vi "Initialize Transfer Groups.vi"(8 "error in (no error)":errorcluster, 10 "transfer group configurations":T1[](array[typedef]) {"transfers"."channels"."string offset" format="%d bytes"}, 11 "PXImc Transceiver in":refnum<class "DSF PXImc Transceiver.lvclass">=refnum) -> (0 "error out":errorcluster, 3 "PXImc Transceiver out":refnum<class "DSF PXImc Transceiver.lvclass">)   [LabVIEW 2017, in "DSF Core.lvlib" / "DSF PXImc Transceiver.lvclass"]
uses:
  DSF PXImc Transceiver.lvclass
  Typedefs/DSF Engine Transfer Group Configuration.ctl
  Typedefs/DSF Direction.ctl
  Typedefs/DSF Timing Info.ctl
  Typedefs/DSF Settings Info.ctl
  Typedefs/DSF Engine Transfer Configuration.ctl
  Typedefs/DSF Byte Order.ctl
  Typedefs/DSF Engine Channel Configuration.ctl
  Typedefs/DSF Data Type.ctl
  Typedefs/DSF Timeout Behavior.ctl
  PXImc Group Data.ctl
  PXImc Transfer Data.ctl
  DSF PXImc Transceiver.lvclass/DSF PXImc Transceiver.ctl
  DSF Core.lvlib
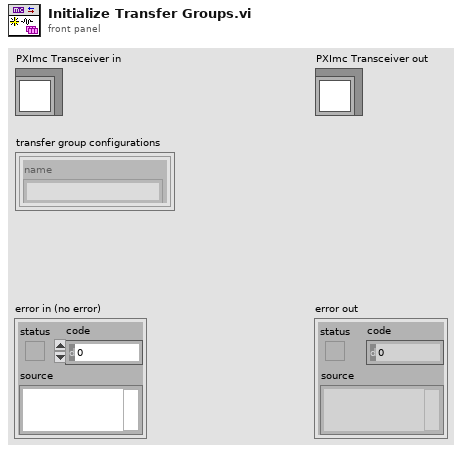
[diagram p1: front panel]
types:
  T1 = typedef "DSF Core.lvlib/DSF Engine Transfer Group Configuration.ctl" = cluster{"name":string, "direction":T2, "cycle timing":T3, "thread index":u8, "settings":T4, "transfers":T5[], "timeout behavior":T9, "convert buffers":bool}
  T2 = typedef "DSF Core.lvlib/DSF Direction.ctl" = enum8{"Tx", "Rx"}
  T3 = typedef "DSF Core.lvlib/DSF Timing Info.ctl" = cluster{"priority":u64, "decimation":u64, "offset":u64}
  T4 = typedef "DSF Core.lvlib/DSF Settings Info.ctl" = cluster{"component":string, "name":string, "values":cluster{"key":string, "value":string}[]}[]
  T5 = typedef "DSF Core.lvlib/DSF Engine Transfer Configuration.ctl" = cluster{"name":string, "byte order":T6, "settings":T4, "channels":T7[]}
  T6 = typedef "DSF Core.lvlib/DSF Byte Order.ctl" = enum8{"big-endian", "little-endian"}
  T7 = typedef "DSF Core.lvlib/DSF Engine Channel Configuration.ctl" = cluster{"string offset":u64, "name":string, "units":string, "engine data type":T8, "string data type":T8, "settings":T4}
  T8 = typedef "DSF Core.lvlib/DSF Data Type.ctl" = enum8{"Bool", "SGL", "DBL", "I8", "I16", "I32", "I64", "U8", "U16", "U32", "U64"}
  T9 = typedef "DSF Core.lvlib/DSF Timeout Behavior.ctl" = enum8{"Increment Late Count", "Throw Error"}
  T10 = typedef "DSF Core.lvlib/DSF PXImc Transceiver.lvclass/PXImc Group Data.ctl" = cluster{"direction":T2, "transfers":T11[]}
  T11 = typedef "DSF Core.lvlib/DSF PXImc Transceiver.lvclass/PXImc Transfer Data.ctl" = cluster{"stream id":u16, "session":refnum<k21>, "buffer size":u64}
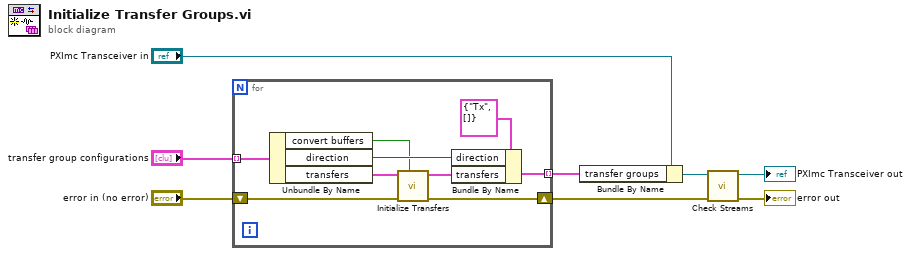
[diagram p0: block diagram]
diagram:
  n1 = for {
    tunnel: "transfer group configurations" -> [w17] mode=indexing
    tunnel: [w9] -> w6 mode=indexing
    shift-right: [w15] -> w4
    shift-left: "error in (no error)" -> [w14]
    n2 = Unbundle By Name(w17) -> ("convert buffers"=w10:bool, "direction"=w11:T2, "transfers"=w12:T5[])
    n3 = call "Initialize Transfers.vi"("enable buffer conversion"=w10, "error in (no error)"=w14, "transfer configurations"=w12) -> ("error out"=w15:errorcluster, "transfers"=w13:T11[])  [unwired: 7 in]
    n4 = Bundle By Name(cluster=T10 {"direction"=enum."Tx", "transfers"=[]} ("PXImc Transfer"), "direction"=w11, "transfers"=w13) -> (w9:T10)
  }
  n5 = Bundle By Name(cluster="PXImc Transceiver in", "transfer groups"=w6) -> (w3:refnum<class "DSF PXImc Transceiver.lvclass">)
  n6 = call "Check Streams.vi"("error in (no error)"=w4, "PXImc Transceiver in"=w3) -> ("error out"=→"error out":errorcluster, "PXImc Transceiver out"=→"PXImc Transceiver out":refnum<class "DSF PXImc Transceiver.lvclass">)  [unwired: 8 in]
